vi "niFpgaGetSimulatedTimeMergeVi.vi"   [LabVIEW 2017]
doc: "Returns the elapsed time of the simulation. For example, you can use this VI to benchmark execution time."
uses:
  <vilib>/FPGA/simulation/niFpgaGetSimulatedTimeNs.vi
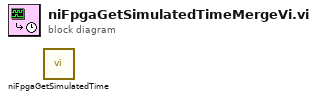
[diagram p0: block diagram]
diagram:
  n1 = call-poly <vilib>:"niFpgaGetSimulatedTime.vi"() -> ()  [unwired: 9 in, 3 out]
